vi "Read Current Command.vi"(8 "error in (no error)":errorcluster, 11 "System Actor in":refnum<class "System Actor.lvclass">) -> (0 "error out":errorcluster, 2 "Current Command":refnum<class "Message Enqueuer.lvclass">, 3 "System Actor out":refnum<class "System Actor.lvclass">)   [LabVIEW 2014, in "Robot Actor Framework.lvlib" / "System Actor.lvlib" / "System Actor.lvclass"]
uses:
  System Actor.lvclass
  <vilib>/ActorFramework/Message Enqueuer/Message Enqueuer.lvclass
  System Actor.lvclass/System Actor.ctl
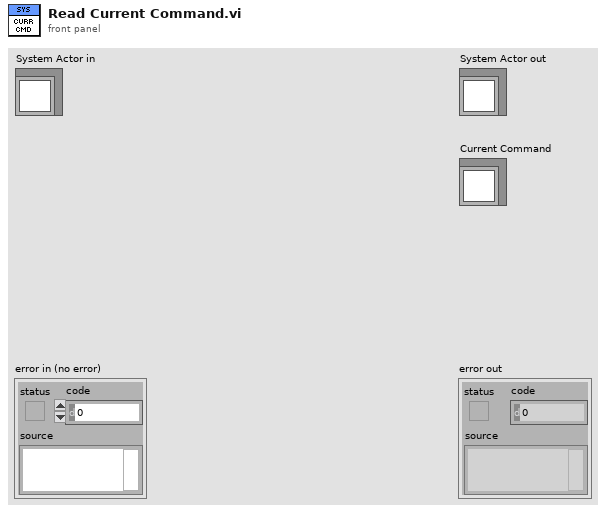
[diagram p1: front panel]
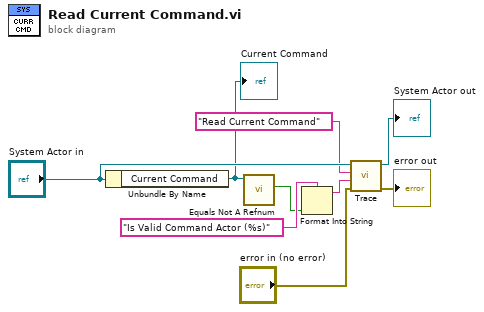
[diagram p0: block diagram]
diagram:
  n1 = Unbundle By Name("System Actor in") -> ("Current Command"=w4:refnum<class "Message Enqueuer.lvclass">)
  "Current Command" <- w4
  n2 = call <vilib>:"Equals Not A Refnum.vi"("Message Enqueuer"=w4) -> ("Not a refnum?"=w2:bool)  [unwired: 10 in]
  n3 = Format Into String(format string="Is Valid Command Actor (%s)", w2) -> (resulting string=w1:string)  [unwired: 2 in, 1 out]
  n4 = call-dynamic "Trace.vi"("error in (no error)"="error in (no error)", "System Message"=w1, "System Action"="Read Current Command", "System Actor in"="System Actor in") -> ("error out"=→"error out":errorcluster, "System Actor out"=→"System Actor out":refnum<class "System Actor.lvclass">)  [unwired: 6 in]
